vi "SubVI_Light Number to String.vi"(11 "Number":u8) -> (3 "String":string)   [LabVIEW 2015]
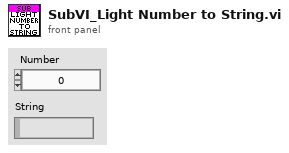
[diagram p1: front panel]
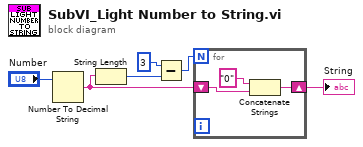
[diagram p0: block diagram]
diagram:
  n1 = Number To Decimal String(number="Number") -> (decimal integer string=w3:string)  [unwired: 1 in]
  n2 = String Length(string=w3) -> (length=w6:i32)
  n3 = Subtract(x=3, y=w6) -> (x-y=w4:i32)
  n4 = for {
    N: w4 -> [_]
    shift-right: [w8] -> w1
    shift-left: w3 -> [w9]
    n5 = Concatenate Strings("0" ("string"), w9) -> (w8:string)
  }
  "String" <- w1
